vi "Move.vi"(8 "error in (no error)":errorcluster, 9 "Absolute (T)":bool=TRUE, 10 "Point":refnum<class "Point.lvclass">, 11 "Rectangle in":refnum<class "Rectangle.lvclass">) -> (0 "error out":errorcluster, 3 "Rectangle out":refnum<class "Rectangle.lvclass">)   [LabVIEW 2021, in "Picture2D.lvlib" / "Rectangle.lvclass"]
uses:
  Rectangle.lvclass
  Shape/Shape.lvclass
  Polygone/Polygone.lvclass
  Point/Point.lvclass
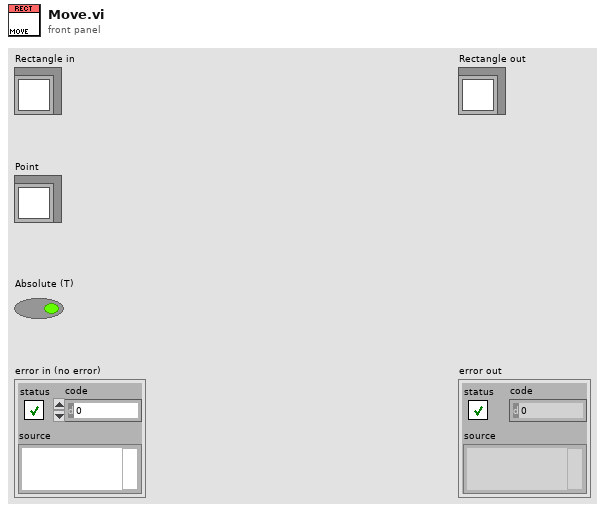
[diagram p1: front panel]
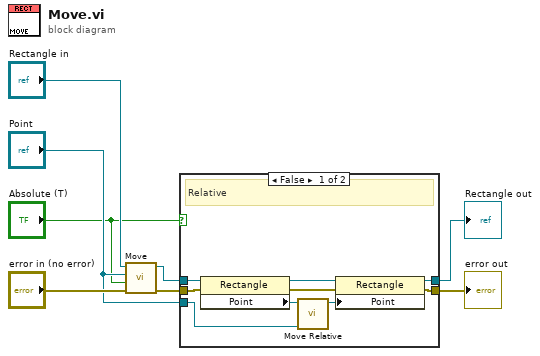
[diagram p0: block diagram]
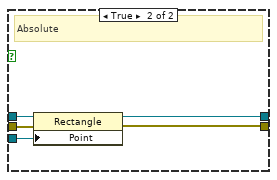
[diagram p2: hidden frame]
diagram:
  n1 = call-parent "Move.vi"("error in (no error)"="error in (no error)", "Absolute (T)"="Absolute (T)", "Point"="Point", "Shape in"="Rectangle in") -> ("error out"=w6:errorcluster, "Shape out"=w3:refnum<class "Rectangle.lvclass">)  [unwired: 6 in]
  n2 = case shown="False" "Absolute (T)" {
    tunnel: w3 -> [w16 w22]
    tunnel: [w12 w21] -> w2
    tunnel: "Point" -> [w17 w20]
    tunnel: w6 -> [w11 w19]
    tunnel: [w9 w18] -> w5
    frame False {
      # "Relative"
      n3 = property class="Rectangle"(reference=w16, error in=w11) -> (reference out=w13:refnum<class "Rectangle.lvclass">, error out=w10:errorcluster, "Point"=w15:refnum<class "Point.lvclass">)
      n4 = call "Move Relative.vi"("Move"=w17, "Point"=w15) -> ("New Point"=w14:refnum<class "Point.lvclass">)  [unwired: 9 in]
      n5 = property class="Rectangle"(reference=w13, error in=w10, "Point"=w14) -> (reference out=w12:refnum<class "Rectangle.lvclass">, error out=w9:errorcluster)
    }
    frame True {
      # "Absolute"
      n6 = property class="Rectangle"(reference=w22, error in=w19, "Point"=w20) -> (reference out=w21:refnum<class "Rectangle.lvclass">, error out=w18:errorcluster)
    }
  }
  "error out" <- w5
  "Rectangle out" <- w2
